vi "actualiza_pot_exc.vi"(3 "Mediciones M in":T1, 4 "Numeric":u32, 5 "Eeprom D-cod M":T3, 6 "COM DATA":T2) -> (0 "set pot":cluster{"Med OUT":dbl, "Nombre":string}, 1 "mediciones M out":T1)   [LabVIEW 2010]
panel:
  out "error out":errorcluster
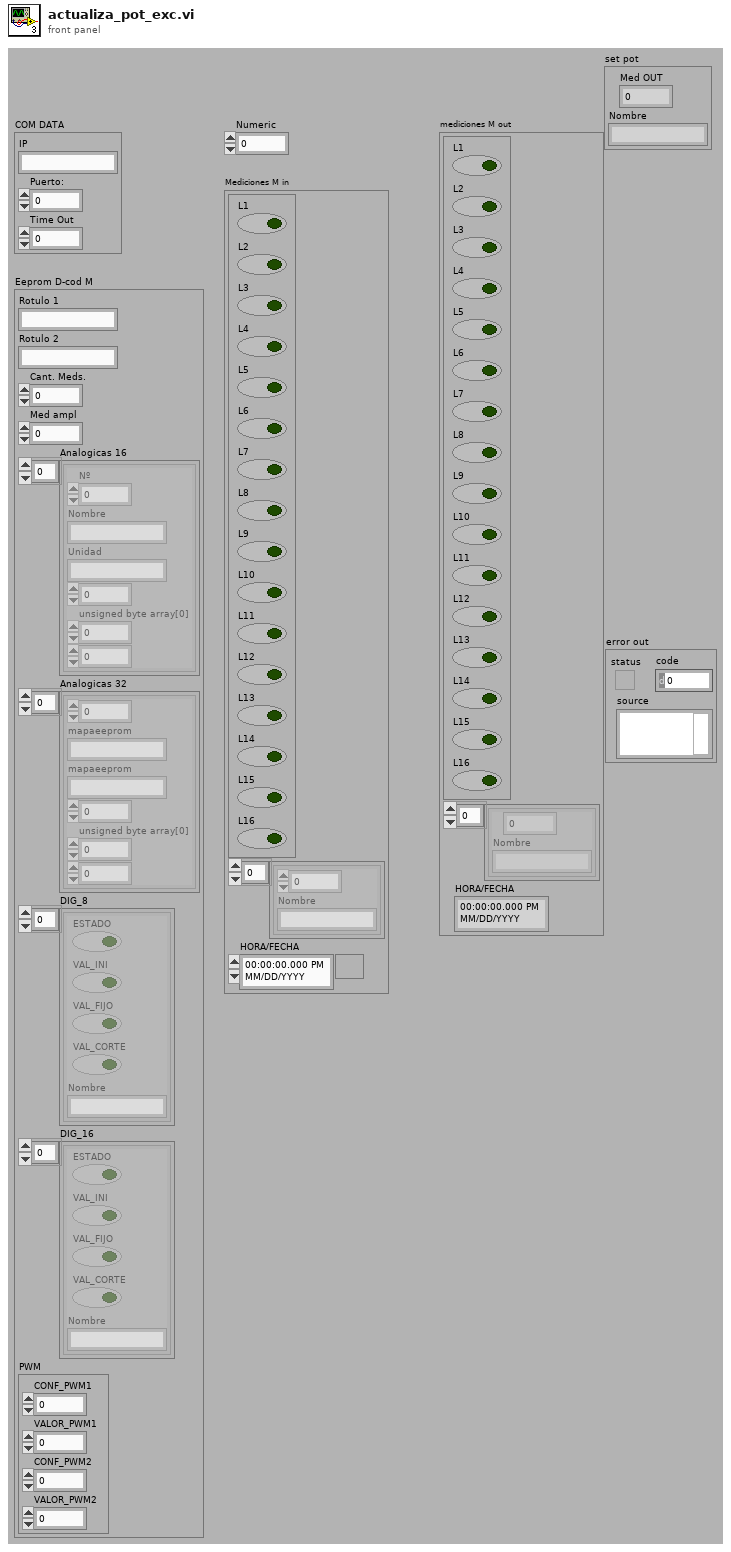
[diagram p1: front panel]
types:
  T1 = cluster{cluster{"L1":bool, "L2":bool, "L3":bool, "L4":bool, "L5":bool, "L6":bool, "L7":bool, "L8":bool, "L9":bool, "L10":bool, "L11":bool, "L12":bool, "L13":bool, "L14":bool, "L15":bool, "L16":bool}, cluster{dbl, "Nombre":string}[], "HORA/FECHA":timestamp}
  T2 = cluster{"IP ":string, "Puerto:":u16, "Time Out":u16}
  T3 = cluster{"Rotulo 1":string, "Rotulo 2":string, "Cant. Meds.":u8, "Med ampl":u8, "Analogicas 16":cluster{"Nº":i32, "Nombre":string, "Unidad":string, u8, "unsigned byte array[0]":u8, u8}[], "Analogicas 32":cluster{i32, "mapaeeprom":string, "mapaeeprom":string, u8, "unsigned byte array[0]":u8, u8}[], "DIG_8":cluster{"ESTADO":bool, "VAL_INI":bool, "VAL_FIJO":bool, "VAL_CORTE":bool, "Nombre":string}[], "DIG_16":cluster{"ESTADO":bool, "VAL_INI":bool, "VAL_FIJO":bool, "VAL_CORTE":bool, "Nombre":string}[], "PWM":cluster{"CONF_PWM1":u8, "VALOR_PWM1":u8, "CONF_PWM2":u8, "VALOR_PWM2":u8}}
  T4 = cluster{i32, "mapaeeprom":string, "mapaeeprom":string, u8, "unsigned byte array[0]":u8, u8}[]
  T5 = cluster{"L1":bool, "L2":bool, "L3":bool, "L4":bool, "L5":bool, "L6":bool, "L7":bool, "L8":bool, "L9":bool, "L10":bool, "L11":bool, "L12":bool, "L13":bool, "L14":bool, "L15":bool, "L16":bool}
  T6 = cluster{i32, "mapaeeprom":string, "mapaeeprom":string, u8, "unsigned byte array[0]":u8, u8}
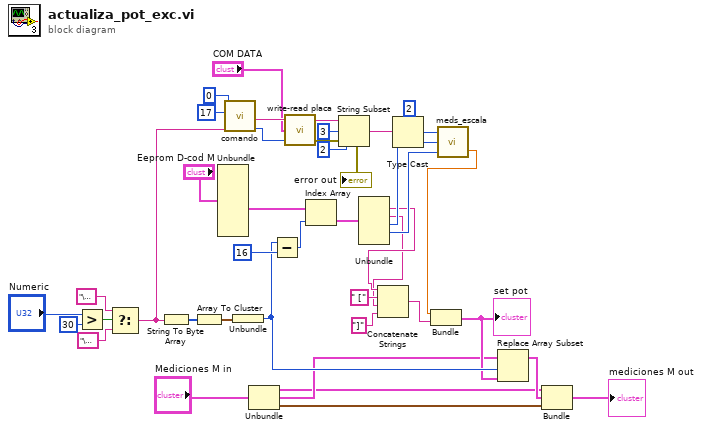
[diagram p0: block diagram]
diagram:
  n1 = Greater?(x="Numeric", y=u32 30) -> (0:w15:bool)
  n2 = Select(t="\u001e" ("LOW"), s=w15, f="\u001a" ("LOW")) -> (s? t:f=w27:string)
  n3 = String To Byte Array(string=w27) -> (unsigned byte array=w28:u8[])
  n4 = Array To Cluster(array=w28) -> (cluster=w29:cluster{"unsigned byte array[0]":u8})
  n5 = Unbundle("Eeprom D-cod M") -> ("Analogicas 32"=w36:T4)  [unwired: 8 out]
  n6 = call "comando.vi"("LOW"=w27, "Comando:"=u8 17, "Equipo Nº"=u8 0) -> ("Bytes OUT"=w18:u16, "comando"=w19:string)  [unwired: 4 in]
  n7 = Unbundle(w29) -> ("unsigned byte array[0]"=w40:u8)
  n8 = Unbundle("Mediciones M in") -> (w11:T5, w31:cluster{dbl, "Nombre":string}[], "HORA/FECHA"=w9:timestamp)
  n9 = Subtract(x=w40, y=u8 16) -> (x-y=w39:u8)
  n10 = call "write-read placa.vi"("Write Command"=w19, "COM DATA"="COM DATA", "bytes"=w18) -> ("LECTURA"=w20:string, "error out"=→"error out":errorcluster)  [unwired: 2 in, 1 out]
  n11 = Index Array(array=w36, index=w39) -> (element=w35:T6)
  n12 = String Subset(string=w20, offset (0)=3, length (rest)=2 ("length (rest)")) -> (substring=w25:string)
  n13 = Unbundle(w35) -> ("mapaeeprom"=w3:string, "mapaeeprom"=w2:string, w37:u8, "unsigned byte array[0]"=w38:u8)  [unwired: 2 out]
  n14 = Concatenate Strings(w3, " [" ("string"), w2, "]" ("string")) -> (w1:string)
  n15 = Type Cast(type=i16 2 ("length (rest)"), x=w25) -> (*(type *) &x=w23:i16)
  n16 = call "meds_escala.vi"("F. Escala"=w38, "linealidad"=w37, "Med IN"=w23) -> ("Med OUT num"=w30:dbl)  [unwired: 1 out]
  n17 = Bundle("Med OUT num"=w30, w1) -> (w32:cluster{"Med OUT num":dbl, string})  [unwired: 1 in]
  "set pot" <- w32
  n18 = Replace Array Subset(array=w31, new element=w32, index=w40) -> (w33:cluster{dbl, "Nombre":string}[])
  n19 = Bundle(w11, w33, "HORA/FECHA"=w9) -> (→"mediciones M out":T1)  [unwired: 1 in]
